vi "FdxCmdRxEDEVlControlCvi.vi"(6 "VLDescriptionIn":T2 {"FilterData" format="%x"; "FilterMask" format="%x"; "FilterMode" items=["FDX_RX_VL_FLT_DIS", "FDX_RX_VL_FLT_ENA ", "FDX_RX_VL_FLT_ENA_INV"]; "VerificationMode" items=["FDX_RX_VL_CHECK_ENA_DEFAULT"=65535, "FDX_RX_VL_CHECK_REDMAM"=16, "DX_RX_VL_CHECK_TRAFIC"=8, "FDX_RX_VL_CHECK_FRAMESIZE"=4, "FDX_RX_VL_CHECK_SNINTEG"=2, "FDX_RX_VL_CHECK_INVPAC"=1, "FDX_RX_VL_CHECK_DISA"=0]}, 8 "error in":errorcluster, 9 "VLEDEDescriptionIn":cluster{"EDESourceIndex":u32}, 10 "VLControlIn":T1 {"PayloadMode" items=["FDX_PAYLOAD_FULL", "FDX_PAYLOAD_IP_EXT", "FDX_PAYLOAD_IP", "FDX_PAYLOAD_MAC"]; "EnableMode" items=["FDX_RX_VL_DIS "=0, "FDX_RX_VL_ENA_STAT"=1, "FDX_RX_VL_ENA_CNT "=2, "FDX_RX_VL_ENA_MON_ALL"=3, "FDX_RX_VL_ENA_MON_GOOD"=7, "FDX_RX_VL_ENA_EXT"=4]}, 11 "InstrumentHandle":u32) -> (0 "error out":errorcluster, 3 "InstrumentHandle":u32)   [LabVIEW 2020, in "AIM664LV.lvlib"]
doc: "This function is used to control the operation of an EDE enabled receive VL. This function should only be used for VL Oriented mode operations (not Chronological monitor or recording receive modes)."
uses:
  AIM664LV.lvlib
  AFDX_LibraryAdmin/FdxGlobalDllPath.vi
panel:
  # "Hex"
  # "Hex"
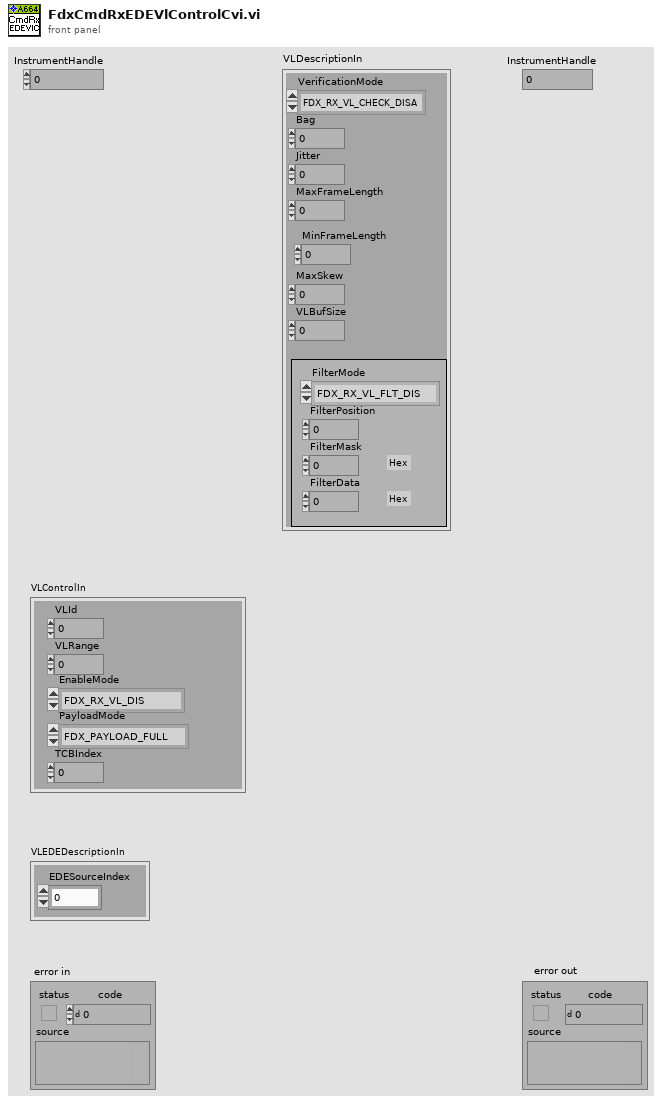
[diagram p1: front panel]
types:
  T1 = cluster{"VLId":u32, "VLRange":u32, "EnableMode":u32, "PayloadMode":u32, "TCBIndex":u32}
  T2 = cluster{"VerificationMode":u32, "Bag":u32, "Jitter":u32, "MaxFrameLength":u32, "MaxSkew":u32, "VLBufSize":u32, "FilterMode":u32, "FilterPosition":u32, "FilterMask":u32, "FilterData":u32, "MinFrameLength":u32}
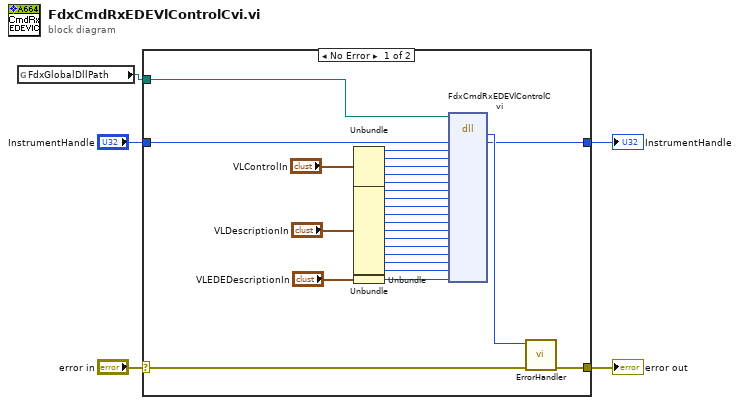
[diagram p0: block diagram]
diagram:
  n1 = global read "FdxGlobalDllPath.vi" "FdxGlobalDllPath"() -> (w3:path)
  n2 = case shown="No Error" "error in" {
    selector: "error in" -> [w30 w33]
    tunnel: [w31 w33] -> w5
    tunnel: w3 -> [w8 _]
    tunnel: "InstrumentHandle" -> [w7 w32]
    tunnel: [w6 w32] -> w1
    frame No Error {
      n3 = Unbundle("VLControlIn") -> ("VLId"=w20:u32, "VLRange"=w21:u32, "EnableMode"=w22:u32, "PayloadMode"=w10:u32, "TCBIndex"=w9:u32)
      n4 = Unbundle("VLDescriptionIn") -> ("VerificationMode"=w19:u32, "Bag"=w27:u32, "Jitter"=w26:u32, "MaxFrameLength"=w25:u32, "MaxSkew"=w18:u32, "VLBufSize"=w17:u32, "FilterMode"=w16:u32, "FilterPosition"=w15:u32, "FilterMask"=w14:u32, "FilterData"=w13:u32, "MinFrameLength"=w12:u32)
      n5 = Unbundle("VLEDEDescriptionIn") -> ("EDESourceIndex"=w11:u32)
      n6 = dll-call lib="aim_fdx.19.dll" fn="FdxCmdRxEDEVlControlCvi"(path in=w8, "InstrumentHandle"=w7, "VLId"=w20, "VLRange"=w21, "EnableMode"=w22, "PayloadMode"=w10, "TCBIndex"=w9, "VerificationMode"=w19, "Bag"=w27, "Jitter"=w26, "MaxFrameLength"=w25, "MaxSkew"=w18, "VLBufSize"=w17, "FilterMode"=w16, "FilterPosition"=w15, "FilterMask"=w14, "FilterData"=w13, "MinFrameLength"=w12, "EDESourceIndex"=w11) -> ("status"=w29:i32, "InstrumentHandle"=w6:u32)  [unwired: 19 in, 2 out]
      n7 = call "ErrorHandler.vi"("error in"=w30, "AIM Error"=w29) -> ("error out"=w31:errorcluster)  [unwired: 9 in]
    }
    frame Error {
    }
  }
  "error out" <- w5
  "InstrumentHandle" <- w1
